vi "JG_adq.vi"() -> ()   [LabVIEW 2019]
uses:
  <vilib>/Analysis/NI_AALBase.lvlib
panel:
  out "JG":dbl
  out "Mlam":dbl
  out "Qlam":dbl
  out "cmiLFE":dbl
  out "cmi*":dbl
  out "M*ar":dbl
  out "rho*":dbl
  out "Q*":dbl
  out "miar":dbl
  out "TlamK":dbl
  out "PlamA":dbl
  in  "TlamC":dbl[](array[numeric])
  in  "Pb":dbl[](array[numeric])
  in  "Plam":dbl[](array[numeric])
  in  "DPlam":dbl[](array[numeric])
  out "QTlam":bool
  out "QPb":bool
  out "QPlam":bool
  out "QDPlam":bool
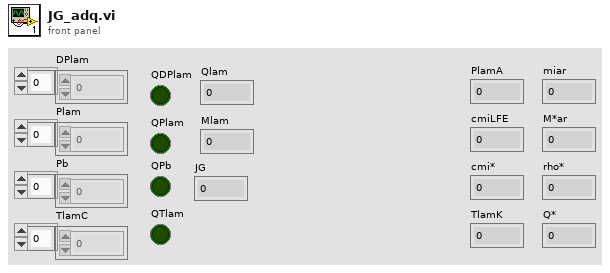
[diagram p1: front panel]
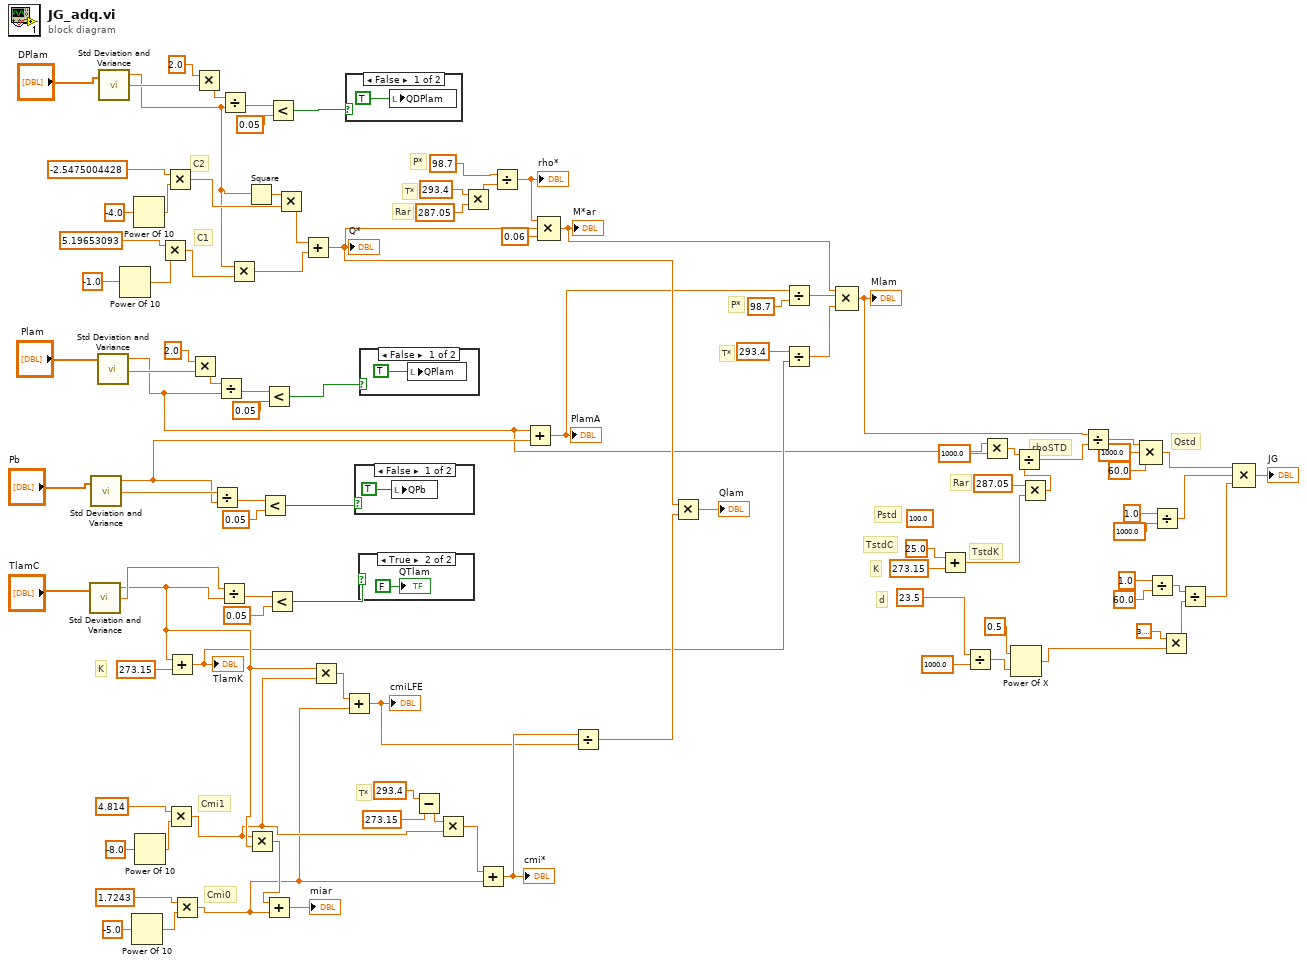
[diagram p0: block diagram]
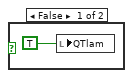
[diagram p2: hidden frame]
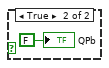
[diagram p3: hidden frame]
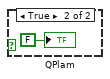
[diagram p4: hidden frame]
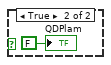
[diagram p5: hidden frame]
diagram:
  (unwired) 100.0
  # "Qstd"
  # "rhoSTD"
  # "K"
  # "Rar"
  # "d"
  # "TstdK"
  # "TstdC"
  # "Pstd"
  # "T*"
  # "P*"
  # "T*"
  # "Rar"
  # "T*"
  # "P*"
  # "C1"
  # "C2"
  # "Cmi0"
  # "Cmi1"
  # "K"
  n1 = call <vilib>:"Std Deviation and Variance.vi"("X"="TlamC") -> ("mean"=w45:dbl, "standard deviation"=w79:dbl)  [unwired: 1 in, 1 out]
  n2 = call <vilib>:"Std Deviation and Variance.vi"("X"="Pb") -> ("mean"=w77:dbl, "standard deviation"=w81:dbl)  [unwired: 1 in, 1 out]
  n3 = call <vilib>:"Std Deviation and Variance.vi"("X"="Plam") -> ("mean"=w27:dbl, "standard deviation"=w95:dbl)  [unwired: 1 in, 1 out]
  n4 = call <vilib>:"Std Deviation and Variance.vi"("X"="DPlam") -> ("mean"=w59:dbl, "standard deviation"=w87:dbl)  [unwired: 1 in, 1 out]
  n5 = Power Of 10(x=-1.0) -> (10^x=w66:dbl)
  n6 = Power Of 10(x=-5.0) -> (10^x=w71:dbl)
  n7 = Power Of 10(x=-4.0) -> (10^x=w64:dbl)
  n8 = Power Of 10(x=-8.0) -> (10^x=w74:dbl)
  n9 = Multiply(x=5.19653093 ("y"), y=w66) -> (x*y=w60:dbl)
  n10 = Multiply(x=-2.5475004428 ("y"), y=w64) -> (x*y=w61:dbl)
  n11 = Multiply(x=4.814 ("y"), y=w74) -> (x*y=w44:dbl)
  n12 = Add(x=w45, y=273.15) -> (x+y=w32:dbl)
  "TlamK" <- w32
  n13 = Multiply(x=1.7243 ("y"), y=w71) -> (x*y=w43:dbl)
  n14 = Multiply(x=2.0, y=w95) -> (x*y=w97:dbl)
  n15 = Multiply(x=2.0, y=w87) -> (x*y=w88:dbl)
  n16 = Divide(x=w81, y=w77) -> (x/y=w84:dbl)
  n17 = Divide(x=w97, y=w27) -> (x/y=w94:dbl)
  n18 = Divide(x=w79, y=w45) -> (x/y=w83:dbl)
  n19 = Divide(x=w88, y=w59) -> (x/y=w90:dbl)
  n20 = Multiply(x=w59, y=w60) -> (x*y=w56:dbl)
  n21 = Square(x=w59) -> (x^2=w58:dbl)
  n22 = Multiply(x=w44, y=w45) -> (x*y=w69:dbl)
  n23 = Less?(x=w84, y=0.05) -> (x < y?=w80:bool)
  n24 = Less?(x=w94, y=0.05) -> (x < y?=w92:bool)
  n25 = Add(x=w69, y=w43) -> (x+y=→"miar":dbl)
  n26 = Less?(x=w83, y=0.05) -> (x < y?=w78:bool)
  n27 = Less?(x=w90, y=0.05) -> (x < y?=w86:bool)
  n28 = Multiply(x=w58, y=w61) -> (x*y=w57:dbl)
  n29 = Add(x=w57, y=w56) -> (x+y=w38:dbl)
  "Q*" <- w38
  n30 = Multiply(x=w45, y=w44) -> (x*y=w42:dbl)
  n31 = Add(x=w42, y=w43) -> (x+y=w40:dbl)
  "cmiLFE" <- w40
  n32 = case shown="False" w86 {
    frame False {
      n33 = local write "QDPlam"(TRUE ("QDPlamLED")) -> ()
    }
    frame True {
      "QDPlam" <- FALSE ("QDPlam")
    }
  }
  n34 = case shown="False" w80 {
    frame False {
      n35 = local write "QPb"(TRUE ("QPbLED")) -> ()
    }
    frame True {
      "QPb" <- FALSE ("QPb")
    }
  }
  n36 = case shown="True" w78 {
    frame False {
      n37 = local write "QTlam"(TRUE ("QTlamLED")) -> ()
    }
    frame True {
      "QTlam" <- FALSE ("QTlam")
    }
  }
  n38 = case shown="False" w92 {
    frame False {
      n39 = local write "QPlam"(TRUE ("QPlamLED")) -> ()
    }
    frame True {
      "QPlam" <- FALSE ("QPlam")
    }
  }
  n40 = Subtract(x=293.4, y=273.15) -> (x-y=w47:dbl)
  n41 = Multiply(x=w47, y=w44) -> (x*y=w46:dbl)
  n42 = Multiply(x=293.4, y=287.05) -> (x*y=w53:dbl)
  n43 = Add(x=w46, y=w43) -> (x+y=w41:dbl)
  "cmi*" <- w41
  n44 = Divide(x=98.7, y=w53) -> (x/y=w51:dbl)
  "rho*" <- w51
  n45 = Add(x=w27, y=w77) -> (x+y=w34:dbl)
  "PlamA" <- w34
  n46 = Compound Arithmetic op=MULTIPLY(w51, w38, 0.06 ("value")) -> (w30:dbl)
  "M*ar" <- w30
  n47 = Divide(x=w41, y=w40) -> (x/y=w39:dbl)
  n48 = Multiply(x=w38, y=w39) -> (x*y=→"Qlam":dbl)
  n49 = Divide(x=w34, y=98.7) -> (x/y=w36:dbl)
  n50 = Divide(x=293.4, y=w32) -> (x/y=w31:dbl)
  n51 = Compound Arithmetic op=MULTIPLY(w30, w36, w31) -> (w17:dbl)
  "Mlam" <- w17
  n52 = Add(x=25.0, y=273.15) -> (x+y=w23:dbl)
  n53 = Divide(x=23.5, y=1000.0) -> (x/y=w6:dbl)
  n54 = Multiply(x=w27, y=1000.0) -> (x*y=w25:dbl)
  n55 = Power Of X(1:w6, 2:0.5 ("y")) -> (0:w4:dbl)
  n56 = Multiply(x=287.05, y=w23) -> (x*y=w22:dbl)
  n57 = Divide(x=w25, y=w22) -> (x/y=w21:dbl)
  n58 = Divide(x=w17, y=w21) -> (x/y=w20:dbl)
  n59 = Compound Arithmetic op=MULTIPLY(w20, 1000.0 ("value"), 60.0 ("value")) -> (w16:dbl)
  n60 = Divide(x=1.0, y=60.0) -> (x/y=w10:dbl)
  n61 = Divide(x=1.0, y=1000.0) -> (x/y=w13:dbl)
  n62 = Multiply(x=3.141592653589793, y=w4) -> (x*y=w3:dbl)
  n63 = Divide(x=w10, y=w3) -> (x/y=w2:dbl)
  n64 = Compound Arithmetic op=MULTIPLY(w16, w13, w2) -> (→"JG":dbl)
